vi "Check URI.vi"(8 "error in (no error)":errorcluster, 10 "Error if invalid (true)":bool=TRUE, 11 "URI":string) -> (0 "error out":errorcluster, 3 "URI":string)   [LabVIEW 2020, in "wamplv.lvlib" / "WAMP Client.lvclass"]
doc: "Check if the URI adherese to the strict WAMP URI standard, with not empty URIs.\n\nOptionally will raise an error if the URI is invalid."
uses:
  WAMP Client.lvclass
  <vilib>/Utility/error.llb/Error Cluster From Error Code.vi
  <vilib>/regexp/Match Regular Expression.xnode
  <vilib>/ErrorRing/Error Ring.xnode
  WAMP Client.lvclass/WAMP Client.ctl
panel:
  out "Valid?":bool
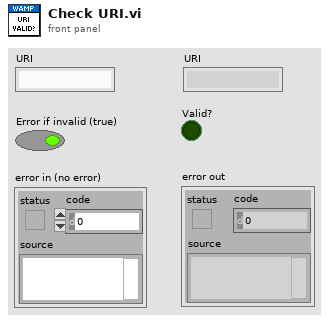
[diagram p1: front panel]
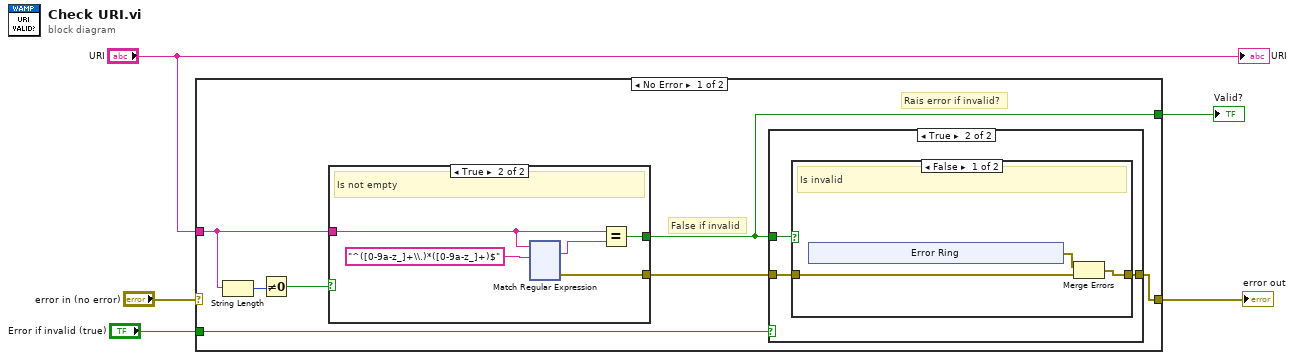
[diagram p0: block diagram]
diagram:
  n1 = case shown="No Error" "error in (no error)" {
    selector: "error in (no error)" -> [_ w145]
    tunnel: [w11 w145] -> w4
    tunnel: "URI" -> [w12 _]
    tunnel: "Error if invalid (true)" -> [w7 _]
    tunnel: [w6 _] -> w1
    frame No Error {
      # "False if invalid"
      # "Rais error if invalid?"
      n2 = String Length(string=w12) -> (length=w8:i32)
      n3 = Not Equal To 0?(x=w8) -> (x != 0?=w9:bool)
      n4 = case shown="True" w9 {
        selector: w9 -> [w25 _]
        tunnel: w12 -> [_ w27]
        tunnel: [w25 w26] -> w6
        tunnel: [_ w29] -> w10
        frame False {
          # "is empty"
        }
        frame True {
          # "Is not empty"
          n5 = xnode "Match Regular Expression"("input string"=w27, "regular expression"="^([0-9a-z_]+\\.)*([0-9a-z_]+)$") -> ("whole match"=w28:string, "error out"=w29:errorcluster)  [unwired: 4 in, 3 out]
          n6 = Equal?(x=w27, y=w28) -> (x = y?=w26:bool)
        }
      }
      n7 = case shown="True" w7 {
        tunnel: w6 -> [_ w16]
        tunnel: [w13 w15] -> w11
        tunnel: w10 -> [w13 w14]
        frame False {
        }
        frame True {
          n8 = case shown="False" w16 {
            tunnel: [w18 w24] -> w15
            tunnel: w14 -> [w17 w24]
            frame False {
              # "Is invalid"
              n9 = xnode "Error Ring"() -> ("error out"=w19:errorcluster)
              n10 = Merge Errors(w19, w17) -> (w18:errorcluster)
            }
            frame True {
              # "is valid"
            }
          }
        }
      }
    }
    frame Error {
    }
  }
  "error out" <- w4
  "Valid?" <- w1
  "URI" <- "URI"
